vi "BRig_Host__Loop_Producer__tcp_System__Data_getExpPrefix_v2.vi"(0 "input_strCmd":string) -> (14 "output_expPrefix_tcp":string, 15 "output_expPrefix_tcp":bool, 16 "output_expPrefix_webdav":string, 17 "output_expPrefix_webdav":bool, 18 "output_expPrefix_any":bool, 19 "output_expPrefix_same":bool)   [LabVIEW 2014]
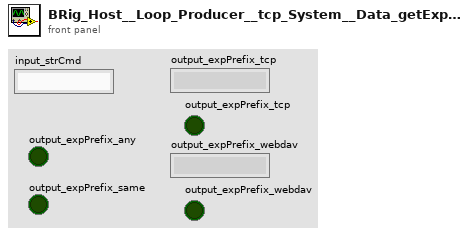
[diagram p1: front panel]
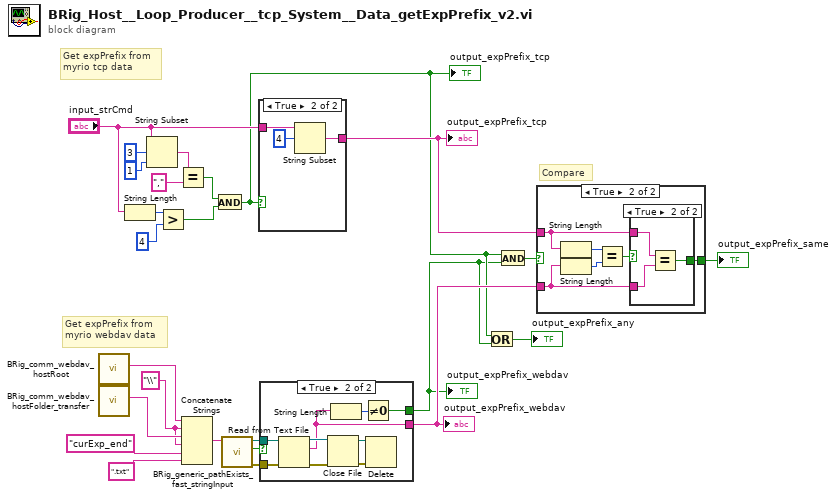
[diagram p0: block diagram]
diagram:
  w19 = "\\" ("string")
  # "Compare"
  # "Get expPrefix from\nmyrio webdav data"
  # "Get expPrefix from\nmyrio tcp data"
  n1 = call "BRig_comm_webdav_hostRoot.vi"() -> ("output_hostRoot"=w20:string)  [unwired: 11 in]
  n2 = call "BRig_comm_webdav_hostFolder_transfer.vi"() -> ("output_HostFolder"=w21:string)  [unwired: 11 in]
  n3 = String Length(string="input_strCmd") -> (length=w11:i32)
  n4 = String Subset(string="input_strCmd", offset (0)=3, length (rest)=1 ("offset (0)")) -> (substring=w23:string)
  n5 = Greater?(x=w11, y=4) -> (0:w8:bool)
  n6 = Equal?(x=w23, y=",") -> (x = y?=w9:bool)
  n7 = Concatenate Strings(w20, w19, w21, w19, "curExp_end" ("intput_fileName"), ".txt" ("string")) -> (w16:string)
  n8 = And(x=w9, y=w8) -> (x .and. y?=w3:bool)
  "output_expPrefix_tcp" <- w3
  n9 = call "BRig_generic_pathExists_fast_stringInput.vi"("input_filePath"=w16) -> ("output_error"=w13:errorcluster, "output_Iexist"=w15:bool, "output_filePath"=w14:path)  [unwired: 8 in]
  n10 = case shown="True" w3 {
    tunnel: "input_strCmd" -> [_ w28]
    tunnel: [_ w26] -> w5
    frame False {
    }
    frame True {
      n11 = String Subset(string=w28, offset (0)=4) -> (substring=w26:string)  [unwired: 1 in]
    }
  }
  "output_expPrefix_tcp" <- w5
  n12 = case shown="True" w15 {
    tunnel: w14 -> [_ w33]
    tunnel: w13 -> [_ w32]
    tunnel: [_ w30] -> w2
    tunnel: [_ w29] -> w6
    frame False {
    }
    frame True {
      n13 = Read from Text File(file (use dialog)=w33, error in=w32) -> (refnum out=w34:refnum<file>, text=w29:string, error out=w35:errorcluster)  [unwired: 2 in, 1 out]
      n14 = Close File(refnum=w34, error in=w35) -> (path=w36:path, error out=w37:errorcluster)
      n15 = String Length(string=w29) -> (length=w31:i32)
      n16 = Not Equal To 0?(x=w31) -> (x != 0?=w30:bool)
      n17 = Delete(path (use dialog)=w36, error in=w37) -> ()  [unwired: 3 in, 3 out]
    }
  }
  "output_expPrefix_webdav" <- w6
  "output_expPrefix_webdav" <- w2
  n18 = Or(x=w3, y=w2) -> (x .or. y?=→"output_expPrefix_any":bool)
  n19 = And(x=w3, y=w2) -> (x .and. y?=w7:bool)
  n20 = case shown="True" w7 {
    tunnel: w6 -> [_ w39]
    tunnel: w5 -> [_ w40]
    tunnel: [_ w38] -> w4
    frame False {
    }
    frame True {
      n21 = String Length(string=w40) -> (length=w43:i32)
      n22 = String Length(string=w39) -> (length=w42:i32)
      n23 = Equal?(x=w43, y=w42) -> (x = y?=w41:bool)
      n24 = case shown="True" w41 {
        tunnel: w40 -> [_ w46]
        tunnel: w39 -> [_ w45]
        tunnel: [_ w44] -> w38
        frame False {
        }
        frame True {
          n25 = Equal?(x=w46, y=w45) -> (x = y?=w44:bool)
        }
      }
    }
  }
  "output_expPrefix_same" <- w4
